vi "Search Component Name.vi"(8 "error in":errorcluster, 10 "Element":string, 11 "Page Refnum":refnum<vi>) -> (0 "error out":errorcluster, 2 "index of element":i32, 3 "Page Refnum":refnum<vi>)   [LabVIEW 2014]
doc: "It search a string element in the Component Name array of the given page in tab control."
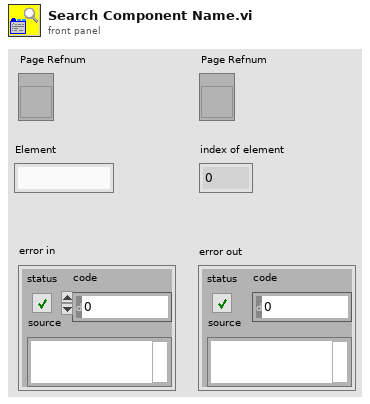
[diagram p1: front panel]
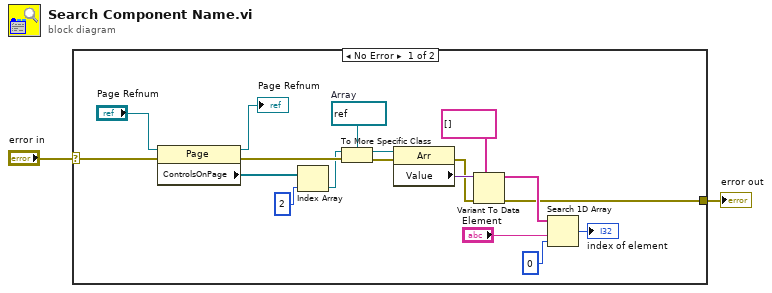
[diagram p0: block diagram]
diagram:
  n1 = case shown="No Error" "error in" {
    selector: "error in" -> [w4 w21]
    tunnel: [w5 w21] -> w2
    frame No Error {
      w15 = refnum<vi> refnum  # Array
      n2 = property class="Page"(reference="Page Refnum", error in=w4) -> (reference out=→"Page Refnum":refnum<vi>, error out=w17:errorcluster, "ControlsOnPage"=w19:refnum<vi>[])
      n3 = Index Array(array=w19, index=2) -> (element=w14:refnum<vi>)
      n4 = To More Specific Class(target class=w15, reference=w14, error in=w17) -> (specific class reference=w13:refnum<vi>, error out=w16:errorcluster)
      n5 = property class="Arr"(reference=w13, error in=w16) -> (error out=w10:errorcluster, "Value"=w11:variant)  [unwired: 1 out]
      n6 = Variant To Data(error in=w10, type=string[] [], Variant=w11) -> (data=w9:string[], error out=w5:errorcluster)
      n7 = Search 1D Array(1D array=w9, element="Element", start index (0)=0) -> (index of element=→"index of element":i32)
    }
    frame Error {
    }
  }
  "error out" <- w2
